vi "Load_Control_subTest.vi"(7 "Test Result in":T2=enum."Success", 8 "error in":errorcluster, 9 "DeviceID":T1, 10 "MicrogridID":u8, 11 "Message Enqueuer in":refnum<class "Message Enqueuer.lvclass">) -> (0 "error out":errorcluster, 1 "dup DeviceID":T1, 2 "dup MicrogridID":u8, 3 "Message Enqueuer out":refnum<class "Message Enqueuer.lvclass">, 5 "Test Result out":T2=enum."Success")   [LabVIEW 2018, in "IED Test Framework.lvlib" / "IED Test.lvclass"]
doc: "This VI tests Activate and Deactive messages as part of DER_Control."
uses:
  IED Test.lvclass
  Controls/Test Result.ctl
  <vilib>/ORNL/CSEISMIC DDS/CSEISMIC DDS Base/Data Types/Controls/DeviceID.ctl
  <vilib>/ActorFramework/Message Enqueuer/Message Enqueuer.lvclass
  <vilib>/ORNL/CSEISMIC DDS/CSEISMIC DDS Base/Data Types/Load_Control.ctl
  <vilib>/ORNL/CSEISMIC DDS/CSEISMIC DDS Base/CSEISMIC DDS.lvclass/CSEISMIC DDS.ctl
  Load Actor/Load Messages/Write Load Control Msg/Write Load Control Msg.lvclass/Write Load Control Msg.ctl
  <vilib>/ActorFramework/Message Enqueuer/Message Enqueuer.lvclass/Message Enqueuer.ctl
  <vilib>/ORNL/CSEISMIC DDS/CSEISMIC DDS Base/Accessors/Write DDS Reference.vi
  <vilib>/ActorFramework/Message Enqueuer/Enqueue.vi
  <vilib>/ORNL/CSEISMIC DDS/CSEISMIC DDS Base/Accessors/Read DDS Reference.vi
  <vilib>/ORNL/CSEISMIC DDS/DDS Reader/DDS Reader.lvclass
  C:/Program Files (x86)/National Instruments/LabVIEW 2018/vi.lib/ORNL/CSEISMIC DDS/CSEISMIC DDS Base/CSEISMIC DDS.lvclass
  Load Actor/Load Messages/Write Load Control Msg/Write Load Control Msg.lvclass
  C:/Program Files (x86)/National Instruments/LabVIEW 2018/vi.lib/ActorFramework/Message/Message.lvclass
  <vilib>/ORNL/CSEISMIC DDS/CSEISMIC DDS Base/Error Handler.vi
  <vilib>/ActorFramework/Message Priority Queue/Priority Enqueue.vi
  <vilib>/ORNL/CSEISMIC DDS/CSEISMIC DDS Base/CSEISMIC DDS.lvclass
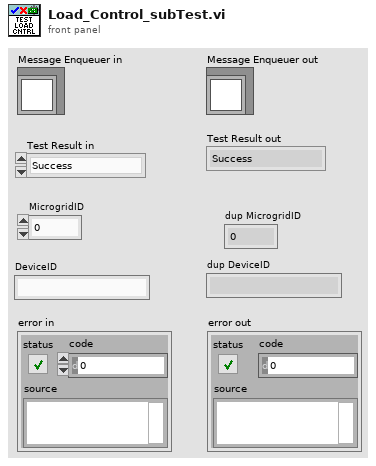
[diagram p1: front panel]
types:
  T1 = typedef "CSEISMIC DDS.lvlib/CSEISMIC DDS.lvclass/DeviceID.ctl" = string
  T2 = typedef "IED Test Framework.lvlib/IED Test.lvclass/Test Result.ctl" = enum16{"Invalid", "Success", "Failure", "Error", "Timeout"}
  T3 = typedef "CSEISMIC DDS.lvlib/CSEISMIC DDS.lvclass/Load_Control.ctl" = cluster{"DeviceID":T1, "Activate":bool, "Deactivate":bool}
  T4 = typedef "LVDDS_library.lvlib/DDS Sample Info.ctl" = cluster{"DDS_SampleStateKind":enum32{"DDS_INVALID_SAMPLE_STATE", "DDS_READ_SAMPLE_STATE", "DDS_NOT_READ_SAMPLE_STATE"}, "DDS_ViewStateKind":enum32{"DDS_INVALID_SAMPLE_STATE", "DDS_NEW_VIEW_STATE", "DDS_NOT_NEW_VIEW_STATE"}, "DDS_InstanceStateKind":enum32{"DDS_INVALID_STATE", "DDS_ALIVE_INSTANCE_STATE", "DDS_NOT_ALIVE_DISPOSED_INSTANCE_STATE", "", "DDS_NOT_ALIVE_NO_WRITERS_INSTANCE_STATE"}, "sec":i32, "nanosec":u32, "valid_data":bool}
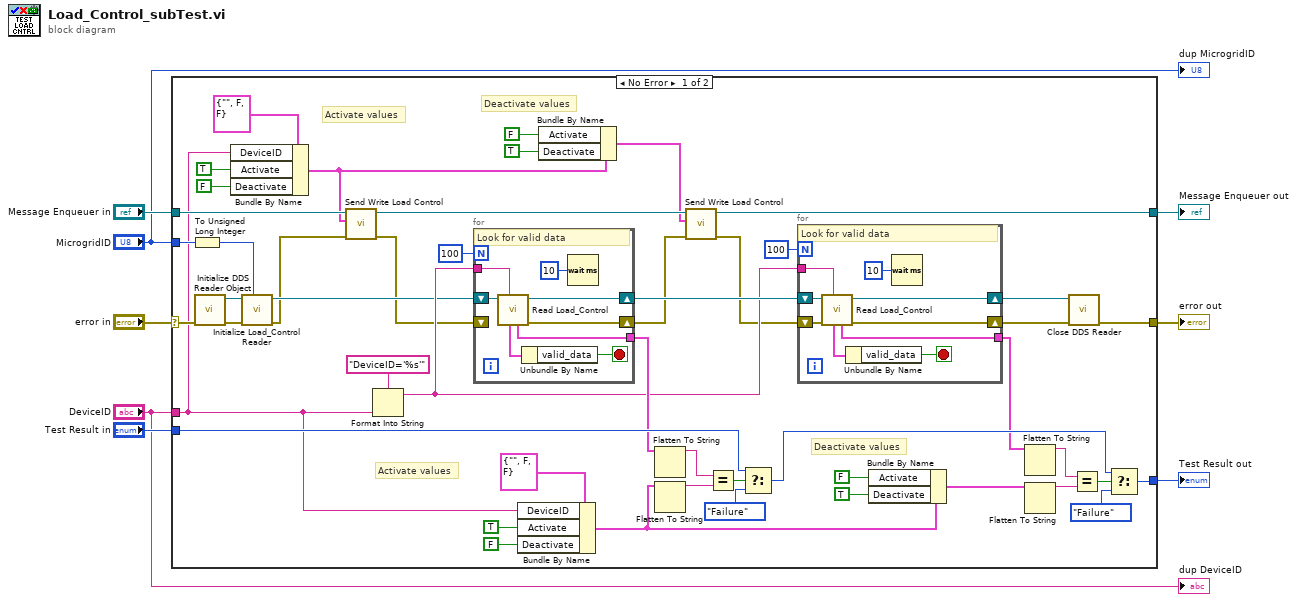
[diagram p0: block diagram]
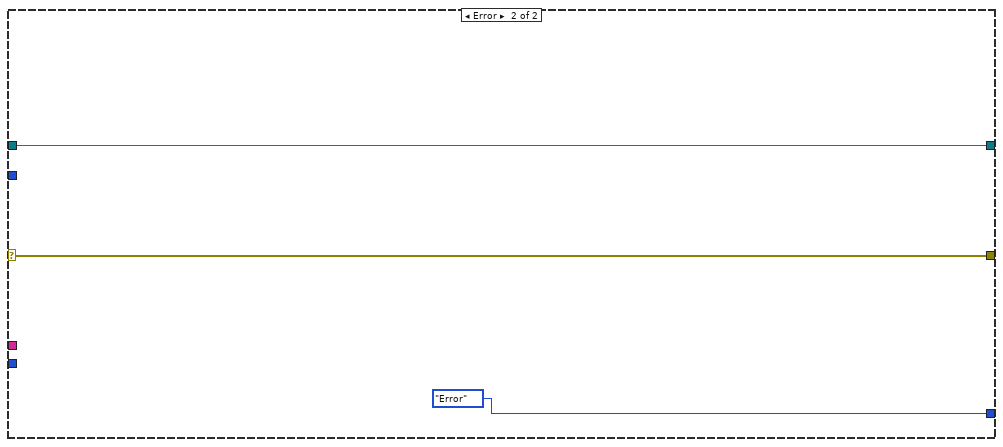
[diagram p2: hidden frame]
diagram:
  n1 = case shown="No Error" "error in" {
    selector: "error in" -> [w44 w76]
    tunnel: [w57 Test_Result."Error" ("Test Result")] -> w1
    tunnel: "DeviceID" -> [w13 _]
    tunnel: [w17 w75] -> w3
    tunnel: "MicrogridID" -> [w43 _]
    tunnel: [w41 w76] -> w2
    tunnel: "Message Enqueuer in" -> [w23 w75]
    tunnel: "Test Result in" -> [w45 _]
    frame No Error {
      # "Deactivate values"
      # "Activate values"
      # "Deactivate values"
      # "Activate values"
      n2 = To Unsigned Long Integer(number=w43) -> (unsigned 32bit integer=w26:u32)
      n3 = call <vilib>:"Initialize DDS Reader Object.vi"("error in"=w44) -> ("error out"=w28:errorcluster, "DDS Reader out"=w27:refnum<class "DDS Reader.lvclass">)  [unwired: 9 in]
      n4 = Bundle By Name(cluster=T3 {"DeviceID"="", "Activate"=FALSE, "Deactivate"=FALSE} ("Load_Control"), "DeviceID"=w13, "Activate"=TRUE, "Deactivate"=FALSE) -> (w10:T3)
      n5 = call <vilib>:"Initialize Load_Control Reader.vi"("MicrogridID"=w26, "error in"=w28, "DDS Reader in"=w27) -> ("error out"=w21:errorcluster, "DDS Reader out"=w25:refnum<class "DDS Reader.lvclass">)  [unwired: 7 in]
      n6 = call "Send Write Load Control.vi"("error in (no error)"=w21, "Load_Control"=w10, "Message Enqueuer"=w23) -> ("error out"=w22:errorcluster, "Message Enqueuer out"=w18:refnum<class "Message Enqueuer.lvclass">)  [unwired: 7 in]
      n7 = Format Into String(format string="DeviceID='%s'", w13) -> (resulting string=w33:string)  [unwired: 2 in, 1 out]
      n8 = for {
        N: 100 -> [_]
        tunnel: [w68] -> w42
        shift-right: [w67] -> w19
        shift-left: w22 -> [_]
        shift-right: [w71] -> w37
        shift-left: w25 -> [w72]
        tunnel: w33 -> [w70]
        stop <- w73 stop-if-true
        # "Look for valid data"
        n9 = call <vilib>:"Read Load_Control.vi"("Query condition"=w70, "DDS Reader in"=w72) -> ("error out"=w67:errorcluster, "DDS Reader out"=w71:refnum<class "DDS Reader.lvclass">, "data"=w68:T3, "DDS Sample Info"=w69:T4)  [unwired: 6 in]
        n10 = Unbundle By Name(w69) -> ("valid_data"=w73:bool)
        n11 = Wait (ms)(milliseconds to wait=u32 10) -> ()  [unwired: 1 out]
      }
      n12 = Bundle By Name(cluster=T3 {"DeviceID"="", "Activate"=FALSE, "Deactivate"=FALSE} ("Load_Control"), "DeviceID"=w13, "Activate"=TRUE, "Deactivate"=FALSE) -> (w30:T3)
      n13 = Bundle By Name(cluster=w10, "Activate"=FALSE, "Deactivate"=TRUE) -> (w9:T3)
      n14 = Flatten To String(anything=w42) -> (data string=w49:string)  [unwired: 3 in, 2 out]
      n15 = Flatten To String(anything=w30) -> (data string=w48:string)  [unwired: 3 in, 2 out]
      n16 = call "Send Write Load Control.vi"("error in (no error)"=w19, "Load_Control"=w9, "Message Enqueuer"=w18) -> ("error out"=w20:errorcluster, "Message Enqueuer out"=w17:refnum<class "Message Enqueuer.lvclass">)  [unwired: 7 in]
      n17 = Equal?(x=w49, y=w48) -> (x = y?=w50:bool)
      n18 = Select(t=w45, s=w50, f=Test_Result."Failure" ("Test Result")) -> (s? t:f=w56:T2)
      n19 = for {
        N: 100 -> [_]
        tunnel: [w63] -> w36
        shift-right: [w65] -> w34
        shift-left: w20 -> [w66]
        shift-right: [w62] -> w35
        shift-left: w37 -> [w64]
        tunnel: w33 -> [w58]
        stop <- w59 stop-if-true
        # "Look for valid data"
        n20 = call <vilib>:"Read Load_Control.vi"("Query condition"=w58, "error in"=w66, "DDS Reader in"=w64) -> ("error out"=w65:errorcluster, "DDS Reader out"=w62:refnum<class "DDS Reader.lvclass">, "data"=w63:T3, "DDS Sample Info"=w60:T4)  [unwired: 5 in]
        n21 = Unbundle By Name(w60) -> ("valid_data"=w59:bool)
        n22 = Wait (ms)(milliseconds to wait=u32 10) -> ()  [unwired: 1 out]
      }
      n23 = Bundle By Name(cluster=w30, "Activate"=FALSE, "Deactivate"=TRUE) -> (w29:T3)
      n24 = Flatten To String(anything=w36) -> (data string=w55:string)  [unwired: 3 in, 2 out]
      n25 = Flatten To String(anything=w29) -> (data string=w54:string)  [unwired: 3 in, 2 out]
      n26 = call <vilib>:"Close DDS Reader.vi"("error in"=w34, "DDS Reader in"=w35) -> ("error out"=w41:errorcluster)  [unwired: 9 in]
      n27 = Equal?(x=w55, y=w54) -> (x = y?=w53:bool)
      n28 = Select(t=w56, s=w53, f=Test_Result."Failure" ("Test Result")) -> (s? t:f=w57:T2)
    }
    frame Error {
    }
  }
  "Test Result out" <- w1
  "Message Enqueuer out" <- w3
  "error out" <- w2
  "dup MicrogridID" <- "MicrogridID"
  "dup DeviceID" <- "DeviceID"
